vi "To BananaLeaf.Assert.vi"(10 "Properties.Assert":refnum<class "Properties.Assert.lvclass">) -> (3 "Leaf.Properties.Assert out":refnum<class "Leaf.Properties.Assert.lvclass">)   [LabVIEW 2021, in "Banana.Caraya.lvlib" / "Leaf.Properties.Assert.lvclass"]
uses:
  Leaf.Properties.Assert.lvclass
  Leaf.Properties.Assert.lvclass/Leaf.Properties.Assert.ctl
  Leaf.Properties/Leaf.Properties.lvclass
  <vilib>/addons/_JKI Toolkits/Caraya/classes/Properties.Assert/Properties.Assert.lvclass
  C:/Program Files (x86)/National Instruments/LabVIEW 2021/vi.lib/addons/_JKI Toolkits/Caraya/classes/Properties/Properties.lvclass
  C:/Program Files (x86)/National Instruments/LabVIEW 2021/vi.lib/addons/_JKI Toolkits/Caraya/classes/Properties.Assert/Properties.Assert.lvclass
  C:/Repositories/LVOS/Bananas/lv-src/Banana.Caraya/Leaf.Properties/Leaf.Properties.lvclass
  C:/Repositories/LVOS/Bananas/lv-src/Bananas/Leaf.Assertion/Leaf.Assertion.lvclass
  C:/Repositories/LVOS/Bananas/lv-src/Bananas/Leaf/Leaf.lvclass
  C:/Repositories/LVOS/Bananas/lv-src/Banana.Caraya/Leaf.Properties.Assert/Leaf.Properties.Assert.lvclass
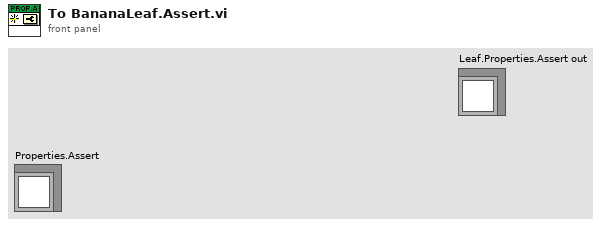
[diagram p1: front panel]
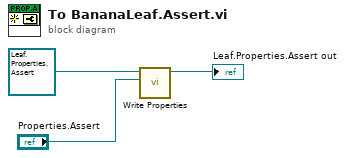
[diagram p0: block diagram]
diagram:
  n1 = call "Write Properties.vi"("Properties"="Properties.Assert", "Leaf.Properties in"=refnum<class "Leaf.Properties.Assert.lvclass"> refnum ("Leaf.Properties.Assert in")) -> ("Leaf.Properties out"=→"Leaf.Properties.Assert out":refnum<class "Leaf.Properties.Assert.lvclass">)  [unwired: 9 in]
